vi "BPG Pressure.vi"(8 "error in (no error)":errorcluster, 10 "BPG Pressure":waveform(dbl), 11 "BPG Pressure in":refnum<class "BPG Pressure.lvclass">) -> (0 "error out":errorcluster, 3 "BPG Pressure out":refnum<class "BPG Pressure.lvclass">)   [LabVIEW 2021, in "BPG Pressure.lvlib" / "BPG Pressure.lvclass"]
uses:
  BPG Pressure.lvclass
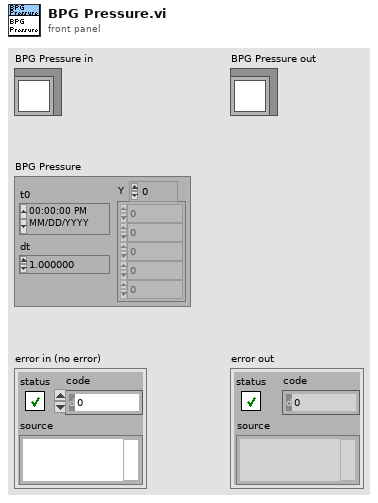
[diagram p1: front panel]
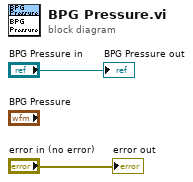
[diagram p0: block diagram]
diagram:
  "error out" <- "error in (no error)"
  "BPG Pressure out" <- "BPG Pressure in"
